vi "UV-VIS Initialize.vi"(3 "error in (no error)":errorcluster, 4 "directory (\"\")":string, 5 "UV-VIS in":refnum<class "CCD_camera.lvclass">) -> (0 "error out":errorcluster, 1 "DLL error code":u32, 2 "Control out":refnum<class "CCD_camera.lvclass">)   [LabVIEW 2019, in "CCD_camera.lvclass"]
doc: "This function will initialize the AndorMCD[tm] System. As part of the initialization procedure the DLL will need access to three files. The first file is \"DETECTOR.INI\" which contains information relating to the detector head, number pixels, readout speeds etc. The second file has the extension \"COF\" and contains the run-time code for the microprocessor on the AndorMCD[tm] plug-in card. The third file has the extension \"RBF\" and contains data for the FPGA on the plug-in card. If \"directory\" is NULL or an empty string then the driver will search the current working directory for the files. If any of these files cannot be loaded then the system will NOT be able to acquire data.\n\n<B>Parameter:</B>\ndirectory - path to the directory containing the files\n\n<B>Error codes:</B>\nDRV_SUCCESS - System fully initialized.\nDRV_VXDNOTINSTALLED - VxD not loaded.\nDRV_INIERROR - Unable to load \"DETECTOR.INI\".\nDRV_COFERROR - Unable to load \"*.COF\".\nDRV_FLEXERROR - Unable to load \"*.RBF\".\nDRV_ERROR_ACK - Unable to communicate with card.\nDRV_ERROR_FILELOAD - Unable to load \"*.COF\" or \"*.RBF\" files.\nDRV_ERROR_PAGELOCK - Unable to acquire lock on requested memory.\n\n<B>NOTES:</B>\n<B>This function must be called first to ensure that the system is fully initialized.</B>"
uses:
  CCD_camera.lvclass
  C:/Users/elysium/Documents/dev/TRANCON/Classes/Detector/Detector.lvclass
  Detector.lvclass/Detector.ctl
  Detector.lvclass
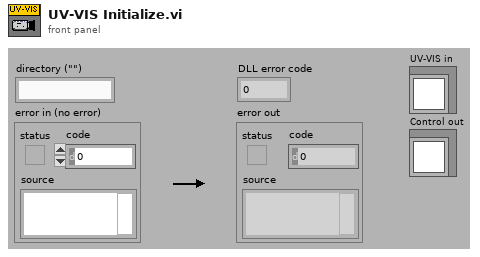
[diagram p1: front panel]
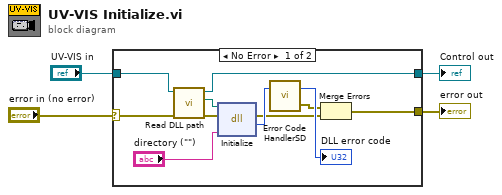
[diagram p0: block diagram]
diagram:
  n1 = case shown="No Error" "error in (no error)" {
    selector: "error in (no error)" -> [w5 w17]
    tunnel: [w11 w17] -> w3
    tunnel: "UV-VIS in" -> [w9 w16]
    tunnel: [w7 w16] -> w1
    frame No Error {
      n2 = call "Read DLL path.vi"("error in (no error)"=w5, "Detector in"=w9) -> ("error out"=w6:errorcluster, "DLL path"=w8:path, "Detector out"=w7:refnum<class "CCD_camera.lvclass">)  [unwired: 7 in]
      n3 = dll-call lib="S:/TRANCON/DLL/Atmcd32d.dll" fn="Initialize"(path in=w8, error in=w6, "directory"="directory (\"\")") -> (error out=w10:errorcluster, "return type"=w15:u32)  [unwired: 2 in, 1 out]
      n4 = call "Error Code HandlerSD.vi"("DLL error code"=w15) -> ("error out"=w12:errorcluster, "dup DLL error code"=→"DLL error code":u32)  [unwired: 1 in]
      n5 = Merge Errors(w12, w10) -> (w11:errorcluster)
    }
    frame Error {
    }
  }
  "error out" <- w3
  "Control out" <- w1
